vi "POST (Buffer).vi"(6 "timeout":i32=10000, 7 "output file":path, 8 "error in":errorcluster, 9 "buffer":string, 10 "url":string, 11 "http-method in":refnum<class "basic-http-client.lvclass">) -> (0 "error out":errorcluster, 2 "response":refnum<class "response.lvclass">, 3 "http-method out":refnum<class "basic-http-client.lvclass">)   [LabVIEW 2020, in "http.lvlib" / "basic-http-client.lvclass"]
uses:
  basic-http-client.lvclass
  response/response.lvclass
  basic-http-client.lvclass/basic-http-client.ctl
  <vilib>/httpClient/POSTBuffer.vi
  <vilib>/httpClient/LabVIEWHTTPClient.lvlib
  http.lvlib
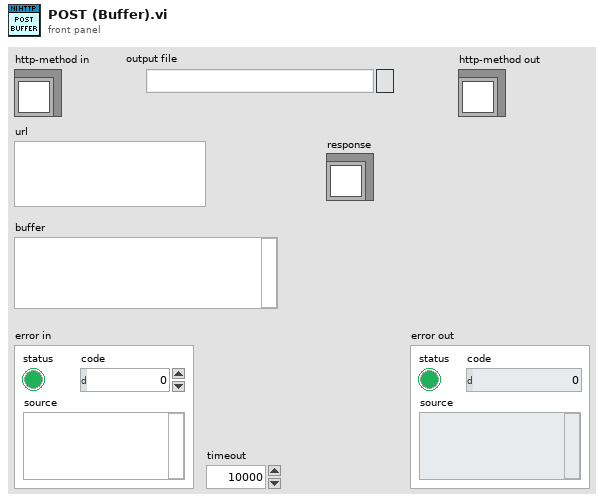
[diagram p1: front panel]
types:
  T1 = typedef "LabVIEWHTTPClient.lvlib/ClientHandle.ctl" = refnum<k1>
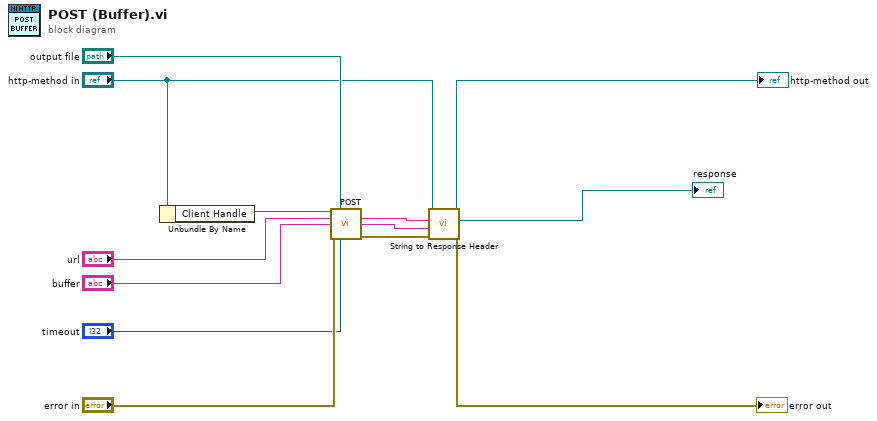
[diagram p0: block diagram]
diagram:
  n1 = Unbundle By Name("http-method in") -> ("Client Handle"=w13:T1)
  n2 = call-poly <vilib>:"POST.vi"("client handle"=w13, "output file"="output file", "url"="url", "buffer"="buffer", "error in (no error)"="error in", "timeout (10000)"="timeout") -> ("headers"=w7:string, "body"=w3:string, "error out"=w6:errorcluster)  [unwired: 6 in, 1 out]
  n3 = call "String to Response Header.vi"("error in (no error)"=w6, "body"=w3, "headers"=w7, "http-client in"="http-method in") -> ("error out"=→"error out":errorcluster, "response"=→"response":refnum<class "response.lvclass">, "http-client out"=→"http-method out":refnum<class "basic-http-client.lvclass">)  [unwired: 5 in]
